vi "Get Actor Core.vi"(8 "error in (no error)":errorcluster, 11 "[V] Waveform in":refnum<class "[V] Waveform.lvclass">) -> (0 "error out":errorcluster, 3 "[V] Waveform out":refnum<class "[V] Waveform.lvclass">)   [LabVIEW 2023, in "[V] Waveform.lvlib" / "[V] Waveform.lvclass"]
uses:
  [V] Waveform.lvclass
  [V] Waveform.lvclass/[V] Waveform.ctl
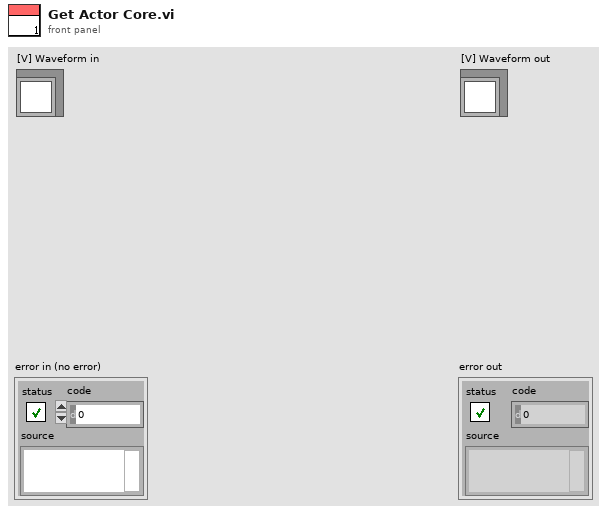
[diagram p1: front panel]
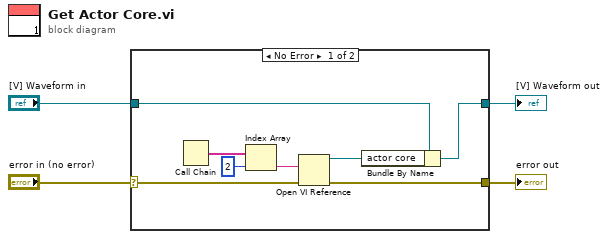
[diagram p0: block diagram]
diagram:
  n1 = case shown="No Error" "error in (no error)" {
    selector: "error in (no error)" -> [w10 w14]
    tunnel: [w5 w14] -> w3
    tunnel: [w6 w13] -> w1
    tunnel: "[V] Waveform in" -> [w8 w13]
    frame No Error {
      n2 = Call Chain() -> (call chain=w12:string[])
      n3 = Index Array(array=w12, index=2) -> (element=w9:string)
      n4 = Open VI Reference(vi path=w9, error in (no error)=w10) -> (vi reference=w7:refnum<vi>, error out=w5:errorcluster)  [unwired: 4 in]
      n5 = Bundle By Name(cluster=w8, "actor core"=w7) -> (w6:refnum<class "[V] Waveform.lvclass">)
    }
    frame Error {
    }
  }
  "error out" <- w3
  "[V] Waveform out" <- w1
